vi "Move new bundler.vi"(6 "Offset":i32=-15, 8 "error in":errorcluster, 9 "New objects created":refnum<vi>[](array[refnum]), 10 "Named Un/Bundler Ref":refnum<vi>, 11 "Tunnel Data Cluster":T1) -> (0 "error out":errorcluster)   [LabVIEW 2023]
doc: "Because a bundler will expand to the right once its labels are set, and we want to place the bundler to the left of a sink terminal, this VI will adjust the new objects created (a bundler and optional constant) to be posisioned the correct offset from the affected terminal. Offset is by default -15px.\n\nThis is not needed for bundlers on source terminals, so we ignore those."
panel:
  out "Move":i32
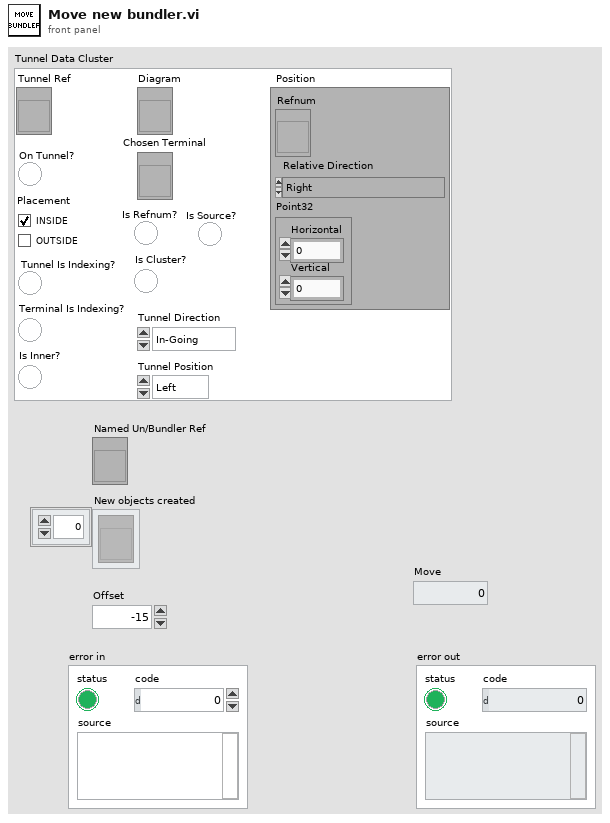
[diagram p1: front panel]
types:
  T1 = cluster{"Tunnel Ref":refnum<vi>, "On Tunnel?":bool, "Placement":enum32{"Choice 1", "Choice 2"}, "Tunnel Is Indexing?":bool, "Diagram":refnum<vi>, "Position":cluster{"Refnum":refnum<vi>, "Relative Direction":enum32{"Right", "Left", "Top", "Bottom", "Top Right", "Top Left", "Bottom Right", "Bottom Left"}, "Point32":cluster{"Horizontal":i32, "Vertical":i32}}, "Chosen Terminal":refnum<vi>, "Is Refnum?":bool, "Is Cluster?":bool, "Is Source?":bool, "Tunnel Direction":enum16{"In-Going", "Out-Going"}, "Tunnel Position":enum16{"Left", "Top", "Right", "Bottom"}, "Is Inner?":bool, "Terminal Is Indexing?":bool}
  T2 = typedef "LVRectTypeDef.ctl" = cluster{"Left":i16, "Top":i16, "Right":i16, "Bottom":i16}
  T3 = typedef "LVPositionTypeDef.ctl" = cluster{"Left":i32, "Top":i32}
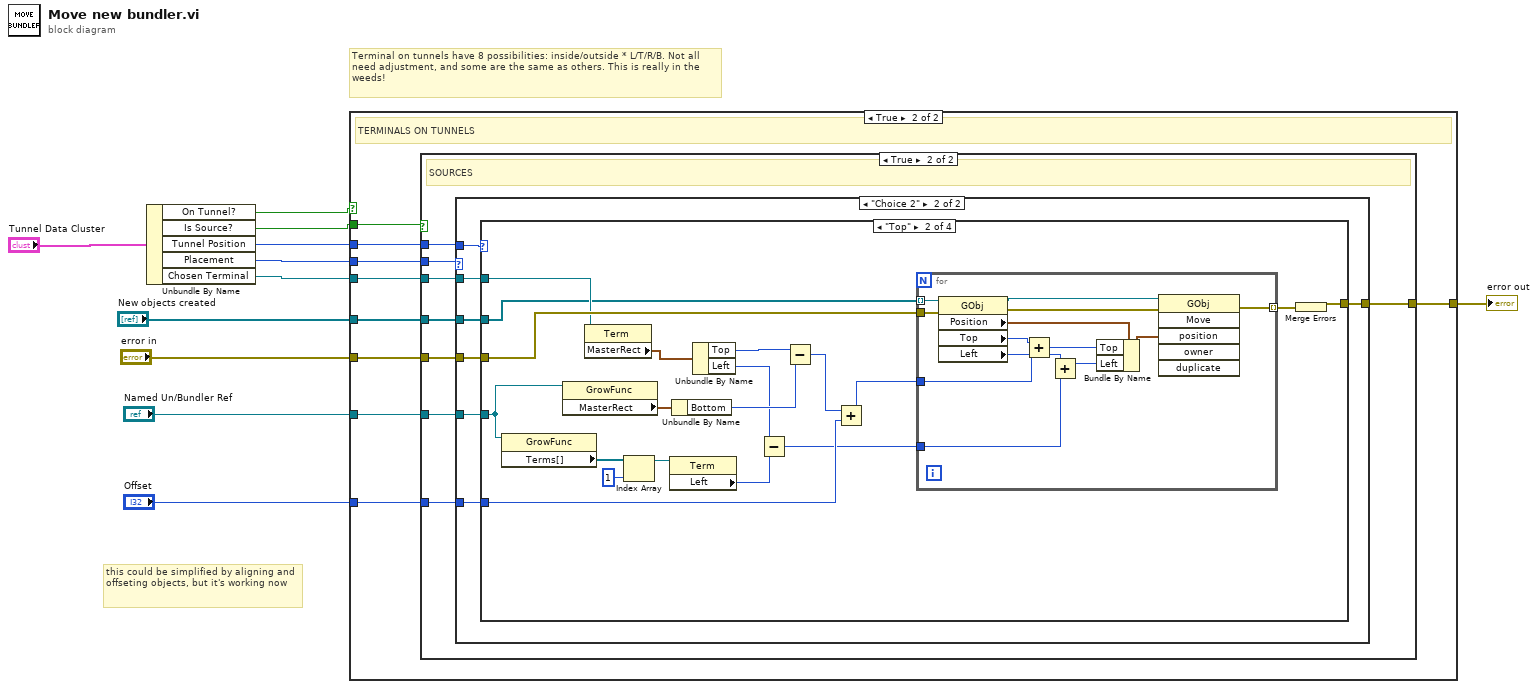
[diagram p0: block diagram]
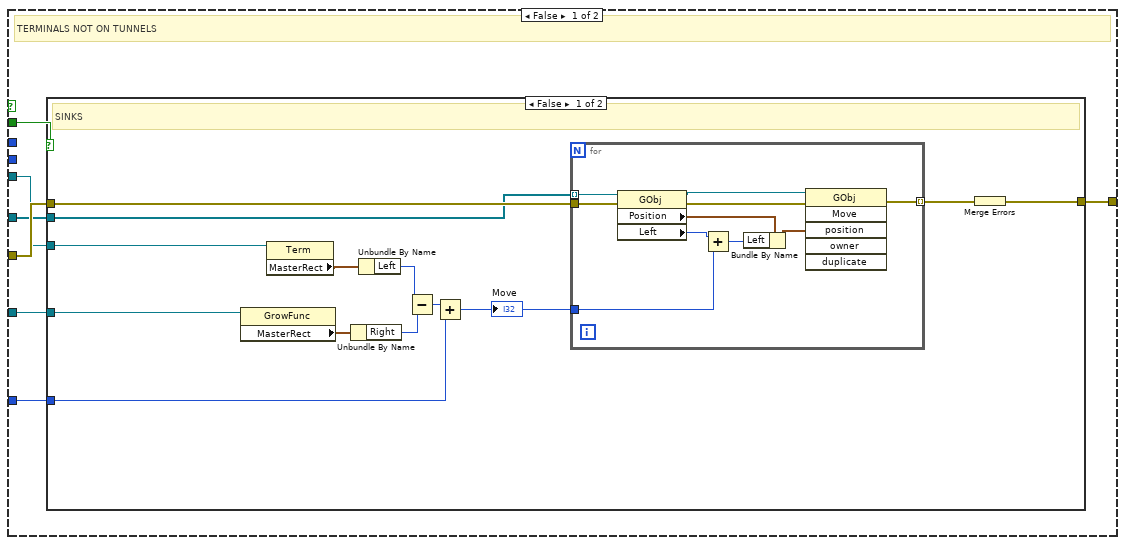
[diagram p2: hidden frame]
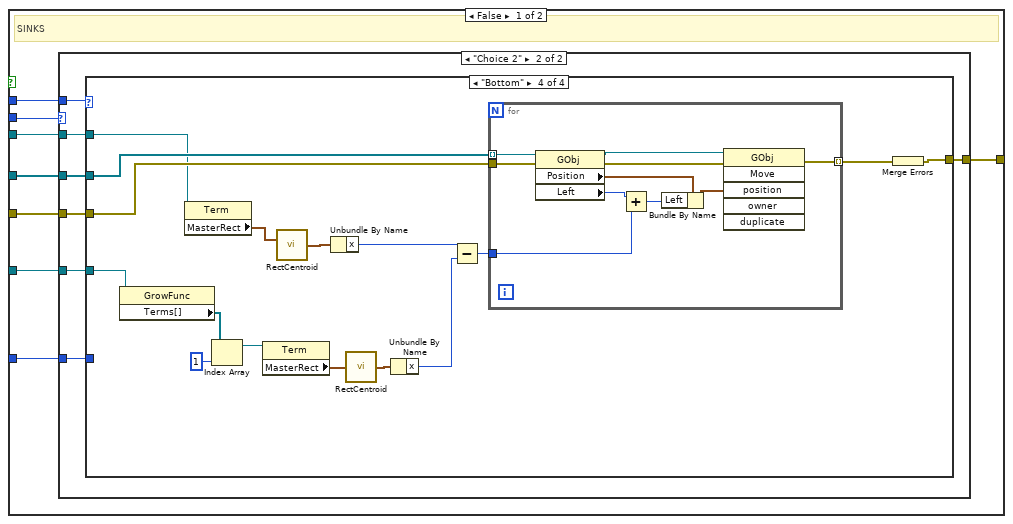
[diagram p4: hidden frame]
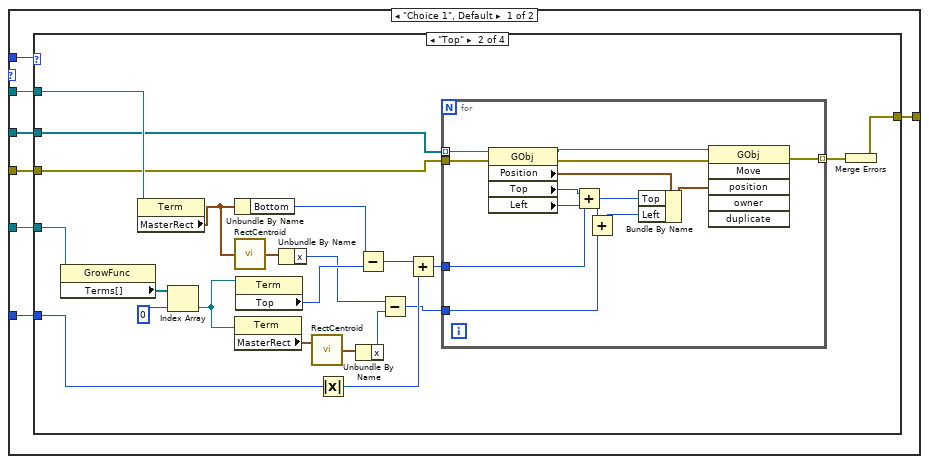
[diagram p5: hidden frame]
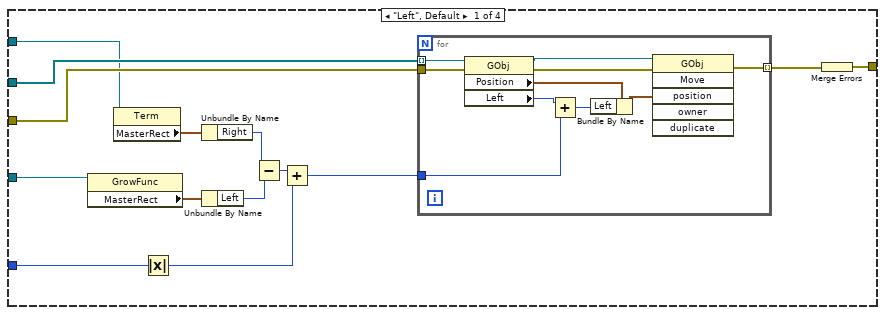
[diagram p6: hidden frame]
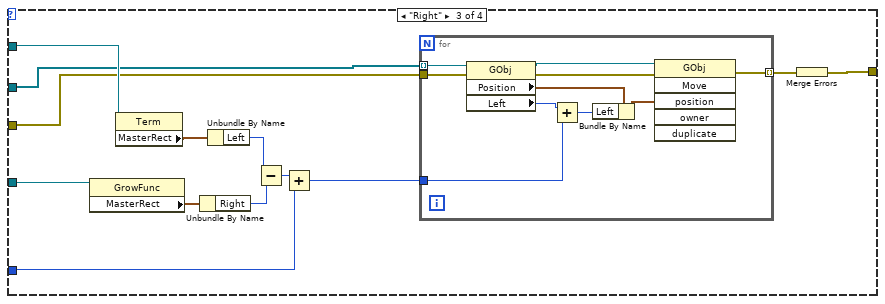
[diagram p7: hidden frame]
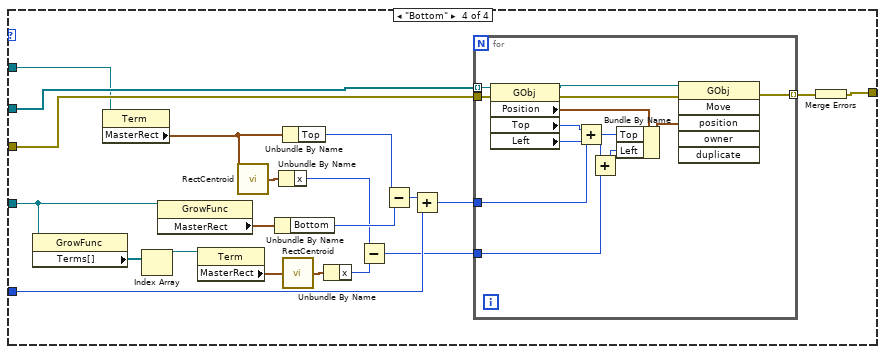
[diagram p8: hidden frame]
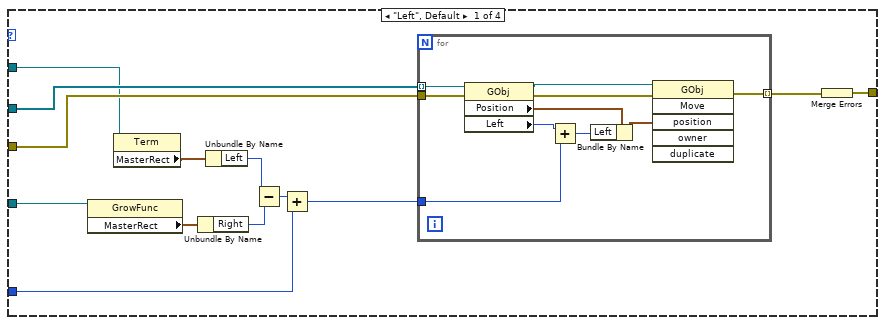
[diagram p9: hidden frame]
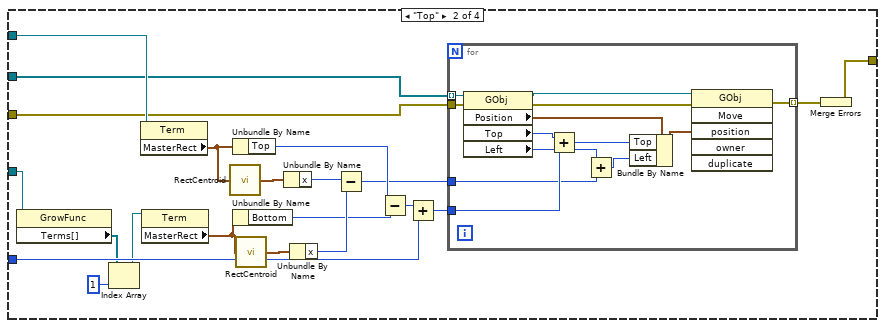
[diagram p10: hidden frame]
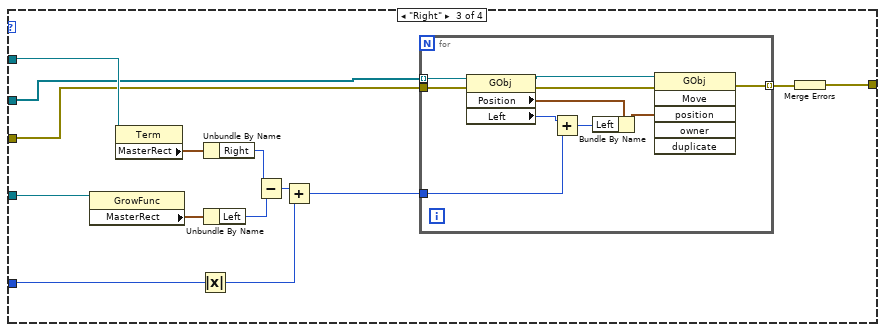
[diagram p11: hidden frame]
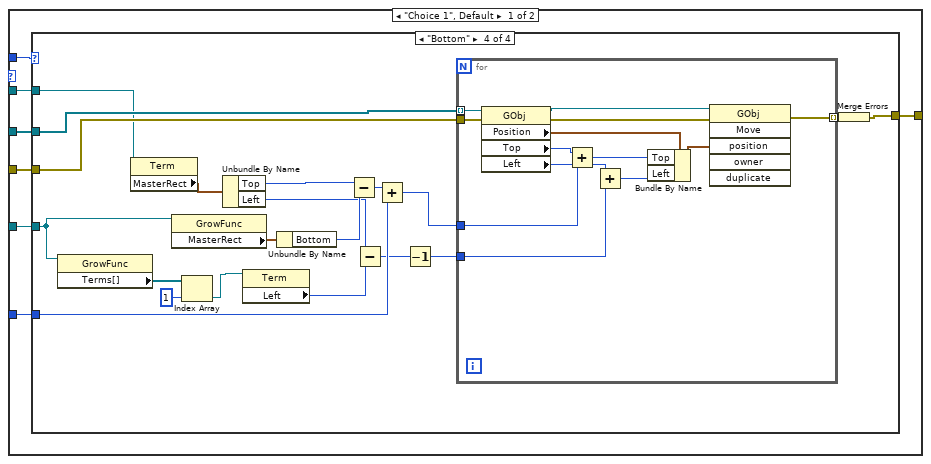
[diagram p12: hidden frame]
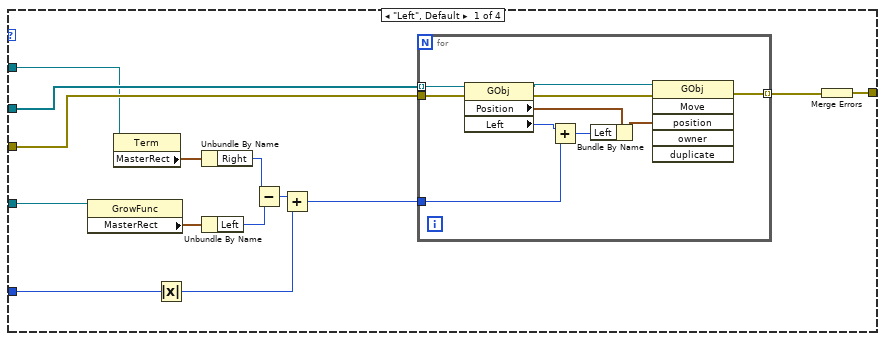
[diagram p13: hidden frame]
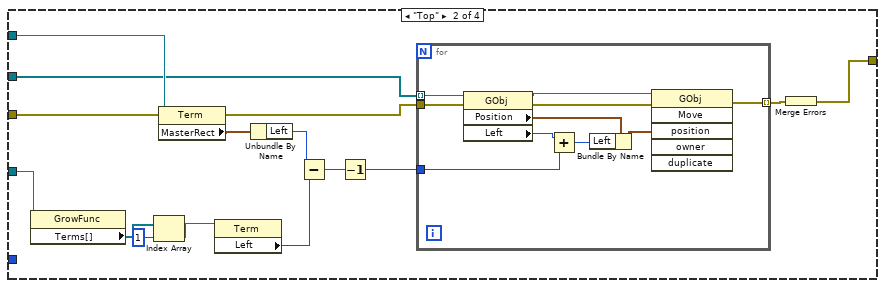
[diagram p14: hidden frame]
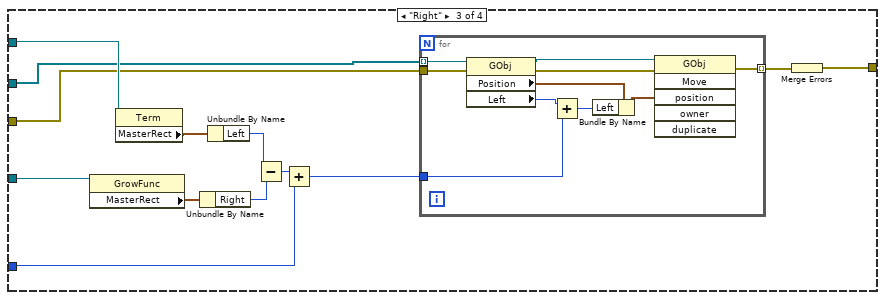
[diagram p15: hidden frame]
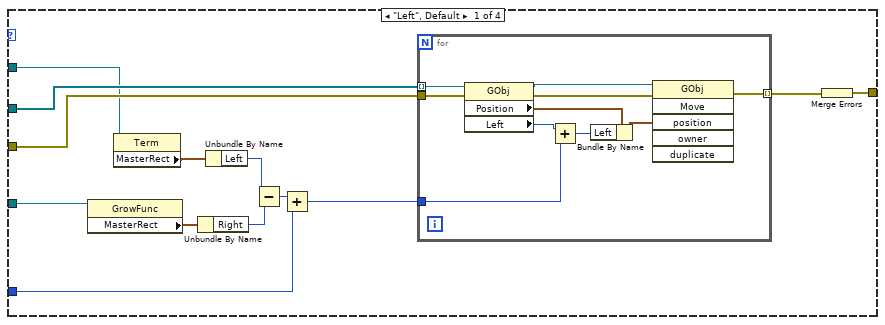
[diagram p16: hidden frame]
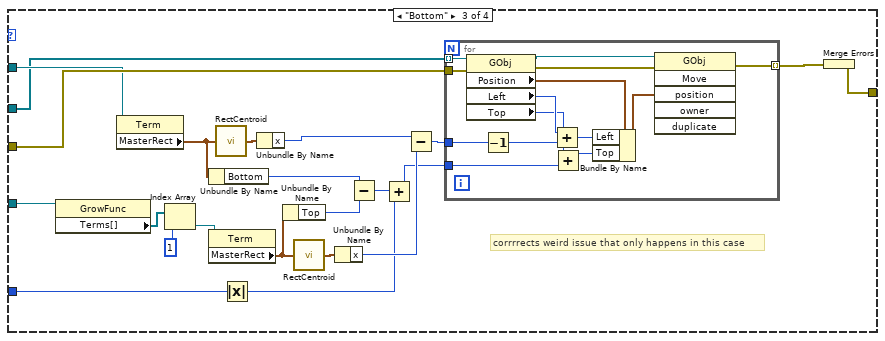
[diagram p17: hidden frame]
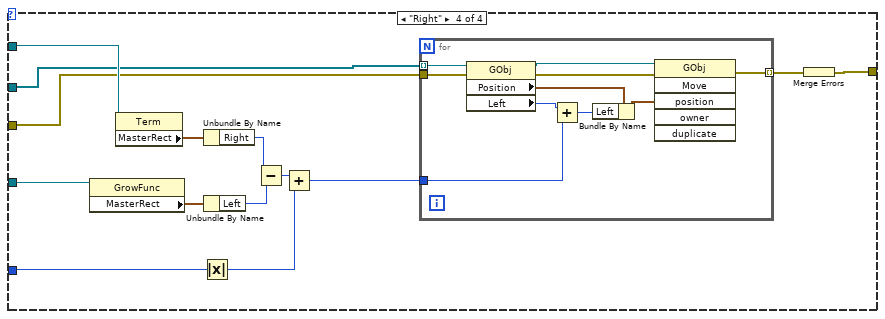
[diagram p18: hidden frame]
diagram:
  # "this could be simplified by aligning and offseting objects, but it's working now"
  # "Terminal on tunnels have 8 possibilities: inside/outside * L/T/R/B. Not all need adjustment, and some are the same as others. This is really in the weeds!"
  n1 = Unbundle By Name("Tunnel Data Cluster") -> ("On Tunnel?"=w5:bool, "Is Source?"=w4:bool, "Tunnel Position"=w3:enum16{"Left", "Top", "Right", "Bottom"}, "Placement"=w2:enum32{"Choice 1", "Choice 2"}, "Chosen Terminal"=w6:refnum<vi>)
  n2 = case shown="True" w5 {
    tunnel: "Offset" -> [w18 w43]
    tunnel: "Named Un/Bundler Ref" -> [w17 w45]
    tunnel: [w16 w48] -> w9
    tunnel: "error in" -> [w15 w47]
    tunnel: w4 -> [w14 w51]
    tunnel: w6 -> [w13 w44]
    tunnel: w3 -> [_ w50]
    tunnel: w2 -> [_ w49]
    tunnel: "New objects created" -> [w12 w46]
    frame False {
      # "TERMINALS NOT ON TUNNELS"
      n3 = case shown="False" w14 {
        tunnel: w18 -> [w30 _]
        tunnel: w17 -> [w29 _]
        tunnel: w13 -> [w27 _]
        tunnel: [w21 w42] -> w16
        tunnel: w15 -> [w20 w42]
        tunnel: w12 -> [w19 _]
        frame False {
          # "SINKS"
          n4 = property class="GrowFunc"(reference=w29) -> ("MasterRect"=w28:T2)  [unwired: 1 in, 2 out]
          n5 = property class="Term"(reference=w27) -> ("MasterRect"=w26:T2)  [unwired: 1 in, 2 out]
          n6 = Unbundle By Name(w28) -> ("Right"=w24:i16)
          n7 = Unbundle By Name(w26) -> ("Left"=w25:i16)
          n8 = Subtract(x=w25, y=w24) -> (x-y=w31:i16)
          n9 = Add(x=w31, y=w30) -> (x+y=w23:i32)
          "Move" <- w23
          n10 = for {
            tunnel: w19 -> [w41] mode=indexing
            tunnel: w23 -> [w38]
            tunnel: w20 -> [w34]
            tunnel: [w32] -> w22 mode=indexing
            n11 = property class="GObj"(reference=w41, error in=w34) -> (reference out=w40:refnum<vi>, error out=w33:errorcluster, "Position"=w37:T3, "Left"=w39:i32)
            n12 = Add(x=w39, y=w38) -> (x+y=w36:i32)
            n13 = Bundle By Name(cluster=w37, "Left"=w36) -> (w35:T3)
            n14 = invoke class="GObj" method="Move"(reference=w40, error in=w33, "position"=w35) -> (error out=w32:errorcluster)  [unwired: 3 in, 5 out]
          }
          n15 = Merge Errors(w22) -> (w21:errorcluster)
        }
        frame True {
          # "these are ok with defaults at palcement time"
          # "SOURCES"
        }
      }
    }
    frame True {
      # "TERMINALS ON TUNNELS"
      n16 = case shown="True" w51 {
        tunnel: w50 -> [w59 w304]
        tunnel: w49 -> [w58 w303]
        tunnel: [w57 w297] -> w48
        tunnel: w47 -> [w56 w300]
        tunnel: w46 -> [w55 w301]
        tunnel: w45 -> [w54 w299]
        tunnel: w44 -> [w53 w302]
        tunnel: w43 -> [w52 w298]
        frame False {
          # "SINKS"
          n17 = case shown="\"Choice 2\"" w58 {
            tunnel: w59 -> [w66 w189]
            tunnel: [w60 w188] -> w57
            tunnel: w56 -> [w63 w187]
            tunnel: w55 -> [w64 w186]
            tunnel: w54 -> [w61 w185]
            tunnel: w53 -> [w65 w184]
            tunnel: w52 -> [w62 w183]
            frame "Choice 1", Default {
              n18 = case shown="\"Top\"" w66 {
                tunnel: [w75 w106 w138 w159] -> w60
                tunnel: w63 -> [w79 w108 w135 w162]
                tunnel: w64 -> [w80 w107 w136 w163]
                tunnel: w61 -> [w78 w105 w134 w158]
                tunnel: w65 -> [w77 w109 w137 w161]
                tunnel: w62 -> [w76 w101 w133 w160]
                frame "Left", Default {
                  n19 = property class="GrowFunc"(reference=w78) -> ("MasterRect"=w73:T2)  [unwired: 1 in, 2 out]
                  n20 = property class="Term"(reference=w77) -> ("MasterRect"=w72:T2)  [unwired: 1 in, 2 out]
                  n21 = Absolute Value(x=w76) -> (abs(x)=w67:i32)
                  n22 = Unbundle By Name(w72) -> ("Right"=w71:i16)
                  n23 = Unbundle By Name(w73) -> ("Left"=w70:i16)
                  n24 = Subtract(x=w71, y=w70) -> (x-y=w74:i16)
                  n25 = Add(x=w74, y=w67) -> (x+y=w69:i32)
                  n26 = for {
                    tunnel: w69 -> [w88]
                    tunnel: [w83] -> w68 mode=indexing
                    tunnel: w80 -> [w82] mode=indexing
                    tunnel: w79 -> [w81]
                    n27 = property class="GObj"(reference=w82, error in=w81) -> (reference out=w90:refnum<vi>, error out=w84:errorcluster, "Position"=w87:T3, "Left"=w89:i32)
                    n28 = Add(x=w89, y=w88) -> (x+y=w86:i32)
                    n29 = Bundle By Name(cluster=w87, "Left"=w86) -> (w85:T3)
                    n30 = invoke class="GObj" method="Move"(reference=w90, error in=w84, "position"=w85) -> (error out=w83:errorcluster)  [unwired: 3 in, 5 out]
                  }
                  n31 = Merge Errors(w68) -> (w75:errorcluster)
                }
                frame "Top" {
                  n32 = property class="GrowFunc"(reference=w105) -> ("Terms[]"=w104:refnum<vi>[])  [unwired: 1 in, 2 out]
                  n33 = property class="Term"(reference=w109) -> ("MasterRect"=w96:T2)  [unwired: 1 in, 2 out]
                  n34 = Index Array(array=w104, index=0) -> (element=w97:refnum<vi>)
                  n35 = Unbundle By Name(w96) -> ("Bottom"=w99:i16)
                  n36 = call <vilib>:"RectCentroid.vi"("rect"=w96) -> ("point"=w95:cluster{"x":i16, "y":i16})
                  n37 = property class="Term"(reference=w97) -> ("MasterRect"=w92:T2)  [unwired: 1 in, 2 out]
                  n38 = property class="Term"(reference=w97) -> ("Top"=w103:i32)  [unwired: 1 in, 2 out]
                  n39 = Unbundle By Name(w95) -> ("x"=w94:i16)
                  n40 = call <vilib>:"RectCentroid.vi"("rect"=w92) -> ("point"=w93:cluster{"x":i16, "y":i16})
                  n41 = Absolute Value(x=w101) -> (abs(x)=w102:i32)
                  n42 = Unbundle By Name(w93) -> ("x"=w91:i16)
                  n43 = Subtract(x=w99, y=w103) -> (x-y=w112:i32)
                  n44 = Subtract(x=w94, y=w91) -> (x-y=w100:i16)
                  n45 = Add(x=w112, y=w102) -> (x+y=w111:i32)
                  n46 = for {
                    tunnel: w111 -> [w123]
                    tunnel: [w118] -> w110 mode=indexing
                    tunnel: w108 -> [w117]
                    tunnel: w107 -> [w116] mode=indexing
                    tunnel: w100 -> [w114]
                    n47 = property class="GObj"(reference=w116, error in=w117) -> (reference out=w125:refnum<vi>, error out=w119:errorcluster, "Position"=w122:T3, "Top"=w124:i32, "Left"=w115:i32)
                    n48 = Add(x=w124, y=w123) -> (x+y=w121:i32)
                    n49 = Add(x=w115, y=w114) -> (x+y=w113:i32)
                    n50 = Bundle By Name(cluster=w122, "Top"=w121, "Left"=w113) -> (w120:T3)
                    n51 = invoke class="GObj" method="Move"(reference=w125, error in=w119, "position"=w120) -> (error out=w118:errorcluster)  [unwired: 3 in, 5 out]
                  }
                  n52 = Merge Errors(w110) -> (w106:errorcluster)
                }
                frame "Right" {
                  n53 = property class="GrowFunc"(reference=w134) -> ("MasterRect"=w131:T2)  [unwired: 1 in, 2 out]
                  n54 = property class="Term"(reference=w137) -> ("MasterRect"=w130:T2)  [unwired: 1 in, 2 out]
                  n55 = Unbundle By Name(w131) -> ("Right"=w128:i16)
                  n56 = Unbundle By Name(w130) -> ("Left"=w129:i16)
                  n57 = Subtract(x=w129, y=w128) -> (x-y=w132:i16)
                  n58 = Add(x=w132, y=w133) -> (x+y=w127:i32)
                  n59 = for {
                    tunnel: w136 -> [w148] mode=indexing
                    tunnel: w127 -> [w145]
                    tunnel: w135 -> [w141]
                    tunnel: [w139] -> w126 mode=indexing
                    n60 = property class="GObj"(reference=w148, error in=w141) -> (reference out=w147:refnum<vi>, error out=w140:errorcluster, "Position"=w144:T3, "Left"=w146:i32)
                    n61 = Add(x=w146, y=w145) -> (x+y=w143:i32)
                    n62 = Bundle By Name(cluster=w144, "Left"=w143) -> (w142:T3)
                    n63 = invoke class="GObj" method="Move"(reference=w147, error in=w140, "position"=w142) -> (error out=w139:errorcluster)  [unwired: 3 in, 5 out]
                  }
                  n64 = Merge Errors(w126) -> (w138:errorcluster)
                }
                frame "Bottom" {
                  n65 = property class="GrowFunc"(reference=w158) -> ("Terms[]"=w157:refnum<vi>[])  [unwired: 1 in, 2 out]
                  n66 = property class="Term"(reference=w161) -> ("MasterRect"=w150:T2)  [unwired: 1 in, 2 out]
                  n67 = Index Array(array=w157) -> (element=w155:refnum<vi>)  [unwired: 1 in]
                  n68 = property class="GrowFunc"(reference=w158) -> ("MasterRect"=w168:T2)  [unwired: 1 in, 2 out]
                  n69 = property class="Term"(reference=w155) -> ("MasterRect"=w154:T2)  [unwired: 1 in, 2 out]
                  n70 = call <vilib>:"RectCentroid.vi"("rect"=w150) -> ("point"=w151:cluster{"x":i16, "y":i16})
                  n71 = Unbundle By Name(w168) -> ("Bottom"=w166:i16)
                  n72 = Unbundle By Name(w151) -> ("x"=w149:i16)
                  n73 = Unbundle By Name(w150) -> ("Top"=w167:i16)
                  n74 = call <vilib>:"RectCentroid.vi"("rect"=w154) -> ("point"=w153:cluster{"x":i16, "y":i16})
                  n75 = Unbundle By Name(w153) -> ("x"=w152:i16)
                  n76 = Subtract(x=w149, y=w152) -> (x-y=w156:i16)
                  n77 = Subtract(x=w167, y=w166) -> (x-y=w169:i16)
                  n78 = Add(x=w169, y=w160) -> (x+y=w165:i32)
                  n79 = for {
                    tunnel: w163 -> [w182] mode=indexing
                    tunnel: w165 -> [w179]
                    tunnel: w162 -> [w175]
                    tunnel: [w173] -> w164 mode=indexing
                    tunnel: w156 -> [w171]
                    n80 = property class="GObj"(reference=w182, error in=w175) -> (reference out=w181:refnum<vi>, error out=w174:errorcluster, "Position"=w178:T3, "Top"=w180:i32, "Left"=w172:i32)
                    n81 = Add(x=w180, y=w179) -> (x+y=w177:i32)
                    n82 = Add(x=w172, y=w171) -> (x+y=w170:i32)
                    n83 = Bundle By Name(cluster=w178, "Top"=w177, "Left"=w170) -> (w176:T3)
                    n84 = invoke class="GObj" method="Move"(reference=w181, error in=w174, "position"=w176) -> (error out=w173:errorcluster)  [unwired: 3 in, 5 out]
                  }
                  n85 = Merge Errors(w164) -> (w159:errorcluster)
                }
              }
            }
            frame "Choice 2" {
              n86 = case shown="\"Bottom\"" w189 {
                tunnel: [w190 w226 w260 w282] -> w188
                tunnel: w187 -> [w194 w228 w257 w284]
                tunnel: w186 -> [w195 w227 w258 w285]
                tunnel: w185 -> [w193 w215 w256 w274]
                tunnel: w184 -> [w192 w229 w259 w283]
                tunnel: w183 -> [w191 w225 w255 _]
                frame "Left", Default {
                  n87 = property class="GrowFunc"(reference=w193) -> ("MasterRect"=w201:T2)  [unwired: 1 in, 2 out]
                  n88 = property class="Term"(reference=w192) -> ("MasterRect"=w200:T2)  [unwired: 1 in, 2 out]
                  n89 = Unbundle By Name(w201) -> ("Right"=w198:i16)
                  n90 = Unbundle By Name(w200) -> ("Left"=w199:i16)
                  n91 = Subtract(x=w199, y=w198) -> (x-y=w202:i16)
                  n92 = Add(x=w202, y=w191) -> (x+y=w197:i32)
                  n93 = for {
                    tunnel: w197 -> [w210]
                    tunnel: [w205] -> w196 mode=indexing
                    tunnel: w195 -> [w204] mode=indexing
                    tunnel: w194 -> [w203]
                    n94 = property class="GObj"(reference=w204, error in=w203) -> (reference out=w212:refnum<vi>, error out=w206:errorcluster, "Position"=w209:T3, "Left"=w211:i32)
                    n95 = Add(x=w211, y=w210) -> (x+y=w208:i32)
                    n96 = Bundle By Name(cluster=w209, "Left"=w208) -> (w207:T3)
                    n97 = invoke class="GObj" method="Move"(reference=w212, error in=w206, "position"=w207) -> (error out=w205:errorcluster)  [unwired: 3 in, 5 out]
                  }
                  n98 = Merge Errors(w196) -> (w190:errorcluster)
                }
                frame "Top" {
                  n99 = property class="GrowFunc"(reference=w215) -> ("Terms[]"=w218:refnum<vi>[])  [unwired: 1 in, 2 out]
                  n100 = Index Array(array=w218, index=1) -> (element=w216:refnum<vi>)
                  n101 = property class="Term"(reference=w229) -> ("MasterRect"=w223:T2)  [unwired: 1 in, 2 out]
                  n102 = property class="Term"(reference=w216) -> ("MasterRect"=w214:T2)  [unwired: 1 in, 2 out]
                  n103 = call <vilib>:"RectCentroid.vi"("rect"=w223) -> ("point"=w224:cluster{"x":i16, "y":i16})
                  n104 = Unbundle By Name(w223) -> ("Top"=w232:i16)
                  n105 = Unbundle By Name(w214) -> ("Bottom"=w213:i16)
                  n106 = call <vilib>:"RectCentroid.vi"("rect"=w214) -> ("point"=w222:cluster{"x":i16, "y":i16})
                  n107 = Unbundle By Name(w224) -> ("x"=w221:i16)
                  n108 = Unbundle By Name(w222) -> ("x"=w220:i16)
                  n109 = Subtract(x=w221, y=w220) -> (x-y=w219:i16)
                  n110 = Subtract(x=w232, y=w213) -> (x-y=w233:i16)
                  n111 = Add(x=w233, y=w225) -> (x+y=w231:i32)
                  n112 = for {
                    tunnel: w231 -> [w244]
                    tunnel: [w239] -> w230 mode=indexing
                    tunnel: w228 -> [w238]
                    tunnel: w227 -> [w237] mode=indexing
                    tunnel: w219 -> [w234]
                    n113 = property class="GObj"(reference=w237, error in=w238) -> (reference out=w246:refnum<vi>, error out=w240:errorcluster, "Position"=w243:T3, "Top"=w245:i32, "Left"=w236:i32)
                    n114 = Add(x=w245, y=w244) -> (x+y=w242:i32)
                    n115 = Add(x=w236, y=w234) -> (x+y=w235:i32)
                    n116 = Bundle By Name(cluster=w243, "Top"=w242, "Left"=w235) -> (w241:T3)
                    n117 = invoke class="GObj" method="Move"(reference=w246, error in=w240, "position"=w241) -> (error out=w239:errorcluster)  [unwired: 3 in, 5 out]
                  }
                  n118 = Merge Errors(w230) -> (w226:errorcluster)
                }
                frame "Right" {
                  n119 = property class="GrowFunc"(reference=w256) -> ("MasterRect"=w253:T2)  [unwired: 1 in, 2 out]
                  n120 = property class="Term"(reference=w259) -> ("MasterRect"=w252:T2)  [unwired: 1 in, 2 out]
                  n121 = Absolute Value(x=w255) -> (abs(x)=w247:i32)
                  n122 = Unbundle By Name(w252) -> ("Right"=w251:i16)
                  n123 = Unbundle By Name(w253) -> ("Left"=w250:i16)
                  n124 = Subtract(x=w251, y=w250) -> (x-y=w254:i16)
                  n125 = Add(x=w254, y=w247) -> (x+y=w249:i32)
                  n126 = for {
                    tunnel: w258 -> [w270] mode=indexing
                    tunnel: w249 -> [w267]
                    tunnel: w257 -> [w263]
                    tunnel: [w261] -> w248 mode=indexing
                    n127 = property class="GObj"(reference=w270, error in=w263) -> (reference out=w269:refnum<vi>, error out=w262:errorcluster, "Position"=w266:T3, "Left"=w268:i32)
                    n128 = Add(x=w268, y=w267) -> (x+y=w265:i32)
                    n129 = Bundle By Name(cluster=w266, "Left"=w265) -> (w264:T3)
                    n130 = invoke class="GObj" method="Move"(reference=w269, error in=w262, "position"=w264) -> (error out=w261:errorcluster)  [unwired: 3 in, 5 out]
                  }
                  n131 = Merge Errors(w248) -> (w260:errorcluster)
                }
                frame "Bottom" {
                  n132 = property class="GrowFunc"(reference=w274) -> ("Terms[]"=w273:refnum<vi>[])  [unwired: 1 in, 2 out]
                  n133 = property class="Term"(reference=w283) -> ("MasterRect"=w278:T2)  [unwired: 1 in, 2 out]
                  n134 = Index Array(array=w273, index=1) -> (element=w271:refnum<vi>)
                  n135 = property class="Term"(reference=w271) -> ("MasterRect"=w279:T2)  [unwired: 1 in, 2 out]
                  n136 = call <vilib>:"RectCentroid.vi"("rect"=w278) -> ("point"=w281:cluster{"x":i16, "y":i16})
                  n137 = Unbundle By Name(w281) -> ("x"=w277:i16)
                  n138 = call <vilib>:"RectCentroid.vi"("rect"=w279) -> ("point"=w280:cluster{"x":i16, "y":i16})
                  n139 = Unbundle By Name(w280) -> ("x"=w276:i16)
                  n140 = Subtract(x=w277, y=w276) -> (x-y=w275:i16)
                  n141 = for {
                    tunnel: w285 -> [w296] mode=indexing
                    tunnel: w284 -> [w290]
                    tunnel: [w288] -> w286 mode=indexing
                    tunnel: w275 -> [w287]
                    n142 = property class="GObj"(reference=w296, error in=w290) -> (reference out=w295:refnum<vi>, error out=w289:errorcluster, "Position"=w293:T3, "Left"=w294:i32)
                    n143 = Add(x=w294, y=w287) -> (x+y=w292:i32)
                    n144 = Bundle By Name(cluster=w293, "Left"=w292) -> (w291:T3)
                    n145 = invoke class="GObj" method="Move"(reference=w295, error in=w289, "position"=w291) -> (error out=w288:errorcluster)  [unwired: 3 in, 5 out]
                  }
                  n146 = Merge Errors(w286) -> (w282:errorcluster)
                }
              }
            }
          }
        }
        frame True {
          # "SOURCES"
          n147 = case shown="\"Choice 2\"" w303 {
            tunnel: w304 -> [w311 w422]
            tunnel: w302 -> [w310 w421]
            tunnel: w301 -> [w309 w420]
            tunnel: w300 -> [w308 w419]
            tunnel: w299 -> [w307 w418]
            tunnel: w298 -> [w306 w417]
            tunnel: [w305 w416] -> w297
            frame "Choice 1", Default {
              n148 = case shown="\"Bottom\"" w311 {
                tunnel: [w320 w346 w372 w391] -> w305
                tunnel: w308 -> [w324 w348 w369 w394]
                tunnel: w309 -> [w325 w347 w370 w395]
                tunnel: w307 -> [w323 w342 w368 w390]
                tunnel: w310 -> [w322 w349 w371 w393]
                tunnel: w306 -> [w321 _ w367 w392]
                frame "Left", Default {
                  n149 = property class="GrowFunc"(reference=w323) -> ("MasterRect"=w318:T2)  [unwired: 1 in, 2 out]
                  n150 = property class="Term"(reference=w322) -> ("MasterRect"=w317:T2)  [unwired: 1 in, 2 out]
                  n151 = Absolute Value(x=w321) -> (abs(x)=w312:i32)
                  n152 = Unbundle By Name(w317) -> ("Right"=w316:i16)
                  n153 = Unbundle By Name(w318) -> ("Left"=w315:i16)
                  n154 = Subtract(x=w316, y=w315) -> (x-y=w319:i16)
                  n155 = Add(x=w319, y=w312) -> (x+y=w314:i32)
                  n156 = for {
                    tunnel: w314 -> [w333]
                    tunnel: [w328] -> w313 mode=indexing
                    tunnel: w325 -> [w327] mode=indexing
                    tunnel: w324 -> [w326]
                    n157 = property class="GObj"(reference=w327, error in=w326) -> (reference out=w335:refnum<vi>, error out=w329:errorcluster, "Position"=w332:T3, "Left"=w334:i32)
                    n158 = Add(x=w334, y=w333) -> (x+y=w331:i32)
                    n159 = Bundle By Name(cluster=w332, "Left"=w331) -> (w330:T3)
                    n160 = invoke class="GObj" method="Move"(reference=w335, error in=w329, "position"=w330) -> (error out=w328:errorcluster)  [unwired: 3 in, 5 out]
                  }
                  n161 = Merge Errors(w313) -> (w320:errorcluster)
                }
                frame "Top" {
                  n162 = property class="GrowFunc"(reference=w342) -> ("Terms[]"=w341:refnum<vi>[])  [unwired: 1 in, 2 out]
                  n163 = Index Array(array=w341, index=1) -> (element=w339:refnum<vi>)
                  n164 = property class="Term"(reference=w349) -> ("MasterRect"=w345:T2)  [unwired: 1 in, 2 out]
                  n165 = property class="Term"(reference=w339) -> ("Left"=w338:i32)  [unwired: 1 in, 2 out]
                  n166 = Unbundle By Name(w345) -> ("Left"=w344:i16)
                  n167 = Subtract(x=w344, y=w338) -> (x-y=w337:i32)
                  n168 = Decrement(x=w337) -> (x-1=w336:i32)
                  n169 = for {
                    tunnel: [w353] -> w343 mode=indexing
                    tunnel: w348 -> [w352]
                    tunnel: w347 -> [w351] mode=indexing
                    tunnel: w336 -> [w350]
                    n170 = property class="GObj"(reference=w351, error in=w352) -> (reference out=w359:refnum<vi>, error out=w354:errorcluster, "Position"=w357:T3, "Left"=w358:i32)
                    n171 = Add(x=w358, y=w350) -> (x+y=w356:i32)
                    n172 = Bundle By Name(cluster=w357, "Left"=w356) -> (w355:T3)
                    n173 = invoke class="GObj" method="Move"(reference=w359, error in=w354, "position"=w355) -> (error out=w353:errorcluster)  [unwired: 3 in, 5 out]
                  }
                  n174 = Merge Errors(w343) -> (w346:errorcluster)
                }
                frame "Right" {
                  n175 = property class="GrowFunc"(reference=w368) -> ("MasterRect"=w365:T2)  [unwired: 1 in, 2 out]
                  n176 = property class="Term"(reference=w371) -> ("MasterRect"=w364:T2)  [unwired: 1 in, 2 out]
                  n177 = Unbundle By Name(w365) -> ("Right"=w362:i16)
                  n178 = Unbundle By Name(w364) -> ("Left"=w363:i16)
                  n179 = Subtract(x=w363, y=w362) -> (x-y=w366:i16)
                  n180 = Add(x=w366, y=w367) -> (x+y=w361:i32)
                  n181 = for {
                    tunnel: w370 -> [w382] mode=indexing
                    tunnel: w361 -> [w379]
                    tunnel: w369 -> [w375]
                    tunnel: [w373] -> w360 mode=indexing
                    n182 = property class="GObj"(reference=w382, error in=w375) -> (reference out=w381:refnum<vi>, error out=w374:errorcluster, "Position"=w378:T3, "Left"=w380:i32)
                    n183 = Add(x=w380, y=w379) -> (x+y=w377:i32)
                    n184 = Bundle By Name(cluster=w378, "Left"=w377) -> (w376:T3)
                    n185 = invoke class="GObj" method="Move"(reference=w381, error in=w374, "position"=w376) -> (error out=w373:errorcluster)  [unwired: 3 in, 5 out]
                  }
                  n186 = Merge Errors(w360) -> (w372:errorcluster)
                }
                frame "Bottom" {
                  n187 = property class="GrowFunc"(reference=w390) -> ("Terms[]"=w389:refnum<vi>[])  [unwired: 1 in, 2 out]
                  n188 = property class="Term"(reference=w393) -> ("MasterRect"=w400:T2)  [unwired: 1 in, 2 out]
                  n189 = property class="GrowFunc"(reference=w390) -> ("MasterRect"=w401:T2)  [unwired: 1 in, 2 out]
                  n190 = Index Array(array=w389, index=1) -> (element=w387:refnum<vi>)
                  n191 = Unbundle By Name(w400) -> ("Top"=w399:i16, "Left"=w386:i16)
                  n192 = property class="Term"(reference=w387) -> ("Left"=w385:i32)  [unwired: 1 in, 2 out]
                  n193 = Unbundle By Name(w401) -> ("Bottom"=w398:i16)
                  n194 = Subtract(x=w399, y=w398) -> (x-y=w402:i16)
                  n195 = Subtract(x=w386, y=w385) -> (x-y=w384:i32)
                  n196 = Add(x=w402, y=w392) -> (x+y=w397:i32)
                  n197 = Decrement(x=w384) -> (x-1=w383:i32)
                  n198 = for {
                    tunnel: w395 -> [w415] mode=indexing
                    tunnel: w397 -> [w412]
                    tunnel: w394 -> [w408]
                    tunnel: [w406] -> w396 mode=indexing
                    tunnel: w383 -> [w403]
                    n199 = property class="GObj"(reference=w415, error in=w408) -> (reference out=w414:refnum<vi>, error out=w407:errorcluster, "Position"=w411:T3, "Top"=w413:i32, "Left"=w405:i32)
                    n200 = Add(x=w413, y=w412) -> (x+y=w410:i32)
                    n201 = Add(x=w405, y=w403) -> (x+y=w404:i32)
                    n202 = Bundle By Name(cluster=w411, "Top"=w410, "Left"=w404) -> (w409:T3)
                    n203 = invoke class="GObj" method="Move"(reference=w414, error in=w407, "position"=w409) -> (error out=w406:errorcluster)  [unwired: 3 in, 5 out]
                  }
                  n204 = Merge Errors(w396) -> (w391:errorcluster)
                }
              }
            }
            frame "Choice 2" {
              n205 = case shown="\"Top\"" w422 {
                tunnel: [w423 w461 w499 w527] -> w416
                tunnel: w419 -> [w427 w460 w497 w524]
                tunnel: w420 -> [w428 w458 w495 w525]
                tunnel: w418 -> [w426 w452 w498 w523]
                tunnel: w421 -> [w425 w459 w496 w526]
                tunnel: w417 -> [w424 w455 w481 w522]
                frame "Left", Default {
                  n206 = property class="GrowFunc"(reference=w426) -> ("MasterRect"=w434:T2)  [unwired: 1 in, 2 out]
                  n207 = property class="Term"(reference=w425) -> ("MasterRect"=w433:T2)  [unwired: 1 in, 2 out]
                  n208 = Unbundle By Name(w434) -> ("Right"=w431:i16)
                  n209 = Unbundle By Name(w433) -> ("Left"=w432:i16)
                  n210 = Subtract(x=w432, y=w431) -> (x-y=w435:i16)
                  n211 = Add(x=w435, y=w424) -> (x+y=w430:i32)
                  n212 = for {
                    tunnel: w430 -> [w443]
                    tunnel: [w438] -> w429 mode=indexing
                    tunnel: w428 -> [w437] mode=indexing
                    tunnel: w427 -> [w436]
                    n213 = property class="GObj"(reference=w437, error in=w436) -> (reference out=w445:refnum<vi>, error out=w439:errorcluster, "Position"=w442:T3, "Left"=w444:i32)
                    n214 = Add(x=w444, y=w443) -> (x+y=w441:i32)
                    n215 = Bundle By Name(cluster=w442, "Left"=w441) -> (w440:T3)
                    n216 = invoke class="GObj" method="Move"(reference=w445, error in=w439, "position"=w440) -> (error out=w438:errorcluster)  [unwired: 3 in, 5 out]
                  }
                  n217 = Merge Errors(w429) -> (w423:errorcluster)
                }
                frame "Top" {
                  n218 = property class="GrowFunc"(reference=w452) -> ("Terms[]"=w451:refnum<vi>[])  [unwired: 1 in, 2 out]
                  n219 = property class="GrowFunc"(reference=w452) -> ("MasterRect"=w454:T2)  [unwired: 1 in, 2 out]
                  n220 = property class="Term"(reference=w459) -> ("MasterRect"=w463:T2)  [unwired: 1 in, 2 out]
                  n221 = Index Array(array=w451, index=1) -> (element=w449:refnum<vi>)
                  n222 = property class="Term"(reference=w449) -> ("Left"=w447:i32)  [unwired: 1 in, 2 out]
                  n223 = Unbundle By Name(w454) -> ("Bottom"=w453:i16)
                  n224 = Unbundle By Name(w463) -> ("Top"=w462:i16, "Left"=w448:i16)
                  n225 = Subtract(x=w448, y=w447) -> (x-y=w446:i32)
                  n226 = Subtract(x=w462, y=w453) -> (x-y=w464:i16)
                  n227 = Add(x=w464, y=w455) -> (x+y=w456:i32)
                  n228 = for {
                    tunnel: w460 -> [w471]
                    tunnel: w458 -> [w470] mode=indexing
                    tunnel: [w469] -> w457 mode=indexing
                    tunnel: w456 -> [w468]
                    tunnel: w446 -> [w465]
                    n229 = property class="GObj"(reference=w470, error in=w471) -> (reference out=w477:refnum<vi>, error out=w472:errorcluster, "Position"=w475:T3, "Top"=w476:i32, "Left"=w467:i32)
                    n230 = Add(x=w476, y=w468) -> (x+y=w474:i32)
                    n231 = Add(x=w467, y=w465) -> (x+y=w466:i32)
                    n232 = Bundle By Name(cluster=w475, "Top"=w474, "Left"=w466) -> (w473:T3)
                    n233 = invoke class="GObj" method="Move"(reference=w477, error in=w472, "position"=w473) -> (error out=w469:errorcluster)  [unwired: 3 in, 5 out]
                  }
                  n234 = Merge Errors(w457) -> (w461:errorcluster)
                }
                frame "Bottom" {
                  # "corrrrects weird issue that only happens in this case"
                  n235 = property class="GrowFunc"(reference=w498) -> ("Terms[]"=w493:refnum<vi>[])  [unwired: 1 in, 2 out]
                  n236 = property class="Term"(reference=w496) -> ("MasterRect"=w485:T2)  [unwired: 1 in, 2 out]
                  n237 = Index Array(array=w493, index=1) -> (element=w490:refnum<vi>)
                  n238 = Unbundle By Name(w485) -> ("Bottom"=w479:i16)
                  n239 = property class="Term"(reference=w490) -> ("MasterRect"=w484:T2)  [unwired: 1 in, 2 out]
                  n240 = call <vilib>:"RectCentroid.vi"("rect"=w485) -> ("point"=w488:cluster{"x":i16, "y":i16})
                  n241 = Absolute Value(x=w481) -> (abs(x)=w478:i32)
                  n242 = Unbundle By Name(w488) -> ("x"=w487:i16)
                  n243 = Unbundle By Name(w484) -> ("Top"=w483:i16)
                  n244 = call <vilib>:"RectCentroid.vi"("rect"=w484) -> ("point"=w491:cluster{"x":i16, "y":i16})
                  n245 = Unbundle By Name(w491) -> ("x"=w489:i16)
                  n246 = Subtract(x=w479, y=w483) -> (x-y=w482:i16)
                  n247 = Add(x=w482, y=w478) -> (x+y=w480:i32)
                  n248 = Subtract(x=w487, y=w489) -> (x-y=w486:i16)
                  n249 = for {
                    tunnel: w497 -> [w507]
                    tunnel: w495 -> [w506] mode=indexing
                    tunnel: [w505] -> w494 mode=indexing
                    tunnel: w486 -> [w504]
                    tunnel: w480 -> [w501]
                    n250 = property class="GObj"(reference=w506, error in=w507) -> (reference out=w513:refnum<vi>, error out=w508:errorcluster, "Position"=w511:T3, "Left"=w512:i32, "Top"=w503:i32)
                    n251 = Decrement(x=w504) -> (x-1=w500:i16)
                    n252 = Add(x=w512, y=w500) -> (x+y=w510:i32)
                    n253 = Add(x=w503, y=w501) -> (x+y=w502:i32)
                    n254 = Bundle By Name(cluster=w511, "Left"=w510, "Top"=w502) -> (w509:T3)
                    n255 = invoke class="GObj" method="Move"(reference=w513, error in=w508, "position"=w509) -> (error out=w505:errorcluster)  [unwired: 3 in, 5 out]
                  }
                  n256 = Merge Errors(w494) -> (w499:errorcluster)
                }
                frame "Right" {
                  n257 = property class="GrowFunc"(reference=w523) -> ("MasterRect"=w520:T2)  [unwired: 1 in, 2 out]
                  n258 = property class="Term"(reference=w526) -> ("MasterRect"=w519:T2)  [unwired: 1 in, 2 out]
                  n259 = Absolute Value(x=w522) -> (abs(x)=w514:i32)
                  n260 = Unbundle By Name(w519) -> ("Right"=w518:i16)
                  n261 = Unbundle By Name(w520) -> ("Left"=w517:i16)
                  n262 = Subtract(x=w518, y=w517) -> (x-y=w521:i16)
                  n263 = Add(x=w521, y=w514) -> (x+y=w516:i32)
                  n264 = for {
                    tunnel: w525 -> [w537] mode=indexing
                    tunnel: w516 -> [w534]
                    tunnel: w524 -> [w530]
                    tunnel: [w528] -> w515 mode=indexing
                    n265 = property class="GObj"(reference=w537, error in=w530) -> (reference out=w536:refnum<vi>, error out=w529:errorcluster, "Position"=w533:T3, "Left"=w535:i32)
                    n266 = Add(x=w535, y=w534) -> (x+y=w532:i32)
                    n267 = Bundle By Name(cluster=w533, "Left"=w532) -> (w531:T3)
                    n268 = invoke class="GObj" method="Move"(reference=w536, error in=w529, "position"=w531) -> (error out=w528:errorcluster)  [unwired: 3 in, 5 out]
                  }
                  n269 = Merge Errors(w515) -> (w527:errorcluster)
                }
              }
            }
          }
        }
      }
    }
  }
  "error out" <- w9
